vi "Terminal Angle Side view int.vi"(0 "Image":T2, 1 "Search Direction ROI 1":u32(ring)=2 items=["Left to Right", "Right to Left", "Top to Bottom", "Bottom to Top"], 5 "ROI Descriptor":T7 {"Contours"."Type" items=["No Selection", "Point", "Line", "Rectangle", "Oval", "Polygon", "Free", "Annulus", "Unused2", "Unused3", "Broken Line", "Free Hand Line", "Rotated Rectangle"]}, 7 "Edge Options ROI 1":T3={"Edge Polarity"=2, "Kernel Size"=5, "Width"=5, "Minimum Edge Strength"=100.0, "Interpolation Type"=enum."Zero Order", "Data Processing Method"=enum."Average"} {"Edge Polarity" items=["All Edges", "Rising Edges", "Falling Edges"]; "Minimum Edge Strength" format="%.2f"; "Width" step=2; "Kernel Size" step=2}, 9 "Line Options ROI 1":T5={"Number of Lines"=1, "Type"=enum."Best Edge Projection", "Min. Score"=10.0, "Max. Score"=1000.0, "Orientation"=0.0, "Angle Range"=10.0, "Angle Tolerance"=1.0, "Step Size"=3, "Min. SNR (db)"=0.0, "Min. Points (%)"=25.0, "Hough Iterations"=5} {"Min. Points (%)" min=0.0 max=100.0; "Min. SNR (db)" min=0.0; "Max. Score" min=0.0 max=1024.0; "Min. Score" min=0.0 max=1024.0 step=1.0}, 11 "error in (no error)":errorcluster, 12 "OverlayOptions":T1) -> (4 "Angle":sgl, 15 "error out":errorcluster)   [LabVIEW 2019, in "Algorithm.lvclass"]
uses:
  FrameworkOverrides/Algorithm.lvclass
  <vilib>/vision/NI_Vision_Development_Module.lvlib
  <vilib>/vision/Measure.llb/Straight Edge Process.ctl
  <vilib>/vision/Measure.llb/Straight Edge Options.ctl
  <vilib>/vision/Measure.llb/Edge Polarity.ctl
  <vilib>/vision/Measure.llb/Edge Options.ctl
  <vilib>/vision/Image Controls.llb/IMAQ Image.ctl
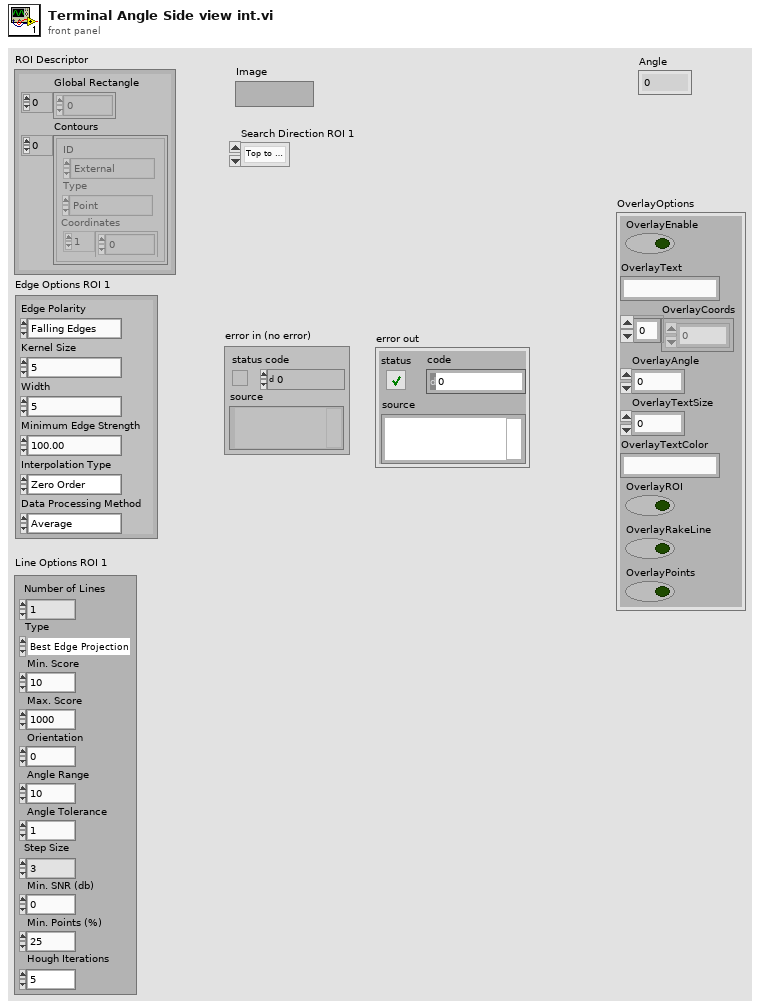
[diagram p1: front panel]
types:
  T1 = cluster{"OverlayEnable":bool, "OverlayText":string, "OverlayCoords":i32[], "OverlayAngle":i32, "OverlayTextSize":i32, "OverlayTextColor":string, "OverlayROI":bool, "OverlayRakeLine":bool, "OverlayPoints":bool}
  T2 = typedef "IMAQ Image.ctl" = refnum<image>
  T3 = typedef "Edge Options.ctl" = cluster{"Edge Polarity":T4, "Kernel Size":u32, "Width":u32, "Minimum Edge Strength":sgl, "Interpolation Type":enum32{"Zero Order", "Bilinear", "Quadratic", "Cubic", "Bilinear Fixed"}, "Data Processing Method":enum32{"Average", "Median"}}
  T4 = typedef "Edge Polarity.ctl" = u32
  T5 = typedef "Straight Edge Options.ctl" = cluster{"Number of Lines":i32, "Type":T6, "Min. Score":dbl, "Max. Score":dbl, "Orientation":dbl, "Angle Range":dbl, "Angle Tolerance":dbl, "Step Size":u32, "Min. SNR (db)":dbl, "Min. Points (%)":dbl, "Hough Iterations":i32}
  T6 = typedef "Straight Edge Process.ctl" = enum32{"First Edge Rake", "Best Edge Rake", "Hough Edge Rake", "First Edge Projection", "Best Edge Projection"}
  T7 = cluster{"Global Rectangle":i32[], "Contours":cluster{"ID":enum32{"External", "Internal"}, "Type":u32, "Coordinates":i32[]}[]}
  T8 = cluster{"Point1 (Pixels)":cluster{"X":sgl, "Y":sgl}, "Point2 (Pixels)":cluster{"X":sgl, "Y":sgl}, "Point1 (Real-World)":cluster{"X":sgl, "Y":sgl}, "Point2 (Real-World)":cluster{"X":sgl, "Y":sgl}, "Angle (Pixel)":dbl, "Angle (Real-World)":dbl, "Score":dbl, "Straightness":dbl, "Average SNR (db)":dbl, "Calibration Valid":bool}[]
  T9 = typedef "Search Line.ctl" = cluster{"Start Point":cluster{"X":sgl, "Y":sgl}, "End Point":cluster{"X":sgl, "Y":sgl}, "Edge Info":T10[], "Edge Map":dbl[], "Calibration Valid":bool}
  T10 = typedef "Edge New.ctl" = cluster{"Location (Pixel)":cluster{"X":sgl, "Y":sgl}, "Location (Real-World)":cluster{"X":sgl, "Y":sgl}, "Distance (Pixel)":dbl, "Distance (Real-World)":dbl, "Strength":dbl, "Noise":dbl, "Rising?":bool}
  T11 = cluster{"Point1 (Pixels)":cluster{"X":sgl, "Y":sgl}, "Point2 (Pixels)":cluster{"X":sgl, "Y":sgl}, "Point1 (Real-World)":cluster{"X":sgl, "Y":sgl}, "Point2 (Real-World)":cluster{"X":sgl, "Y":sgl}, "Angle (Pixel)":dbl, "Angle (Real-World)":dbl, "Score":dbl, "Straightness":dbl, "Average SNR (db)":dbl, "Calibration Valid":bool}
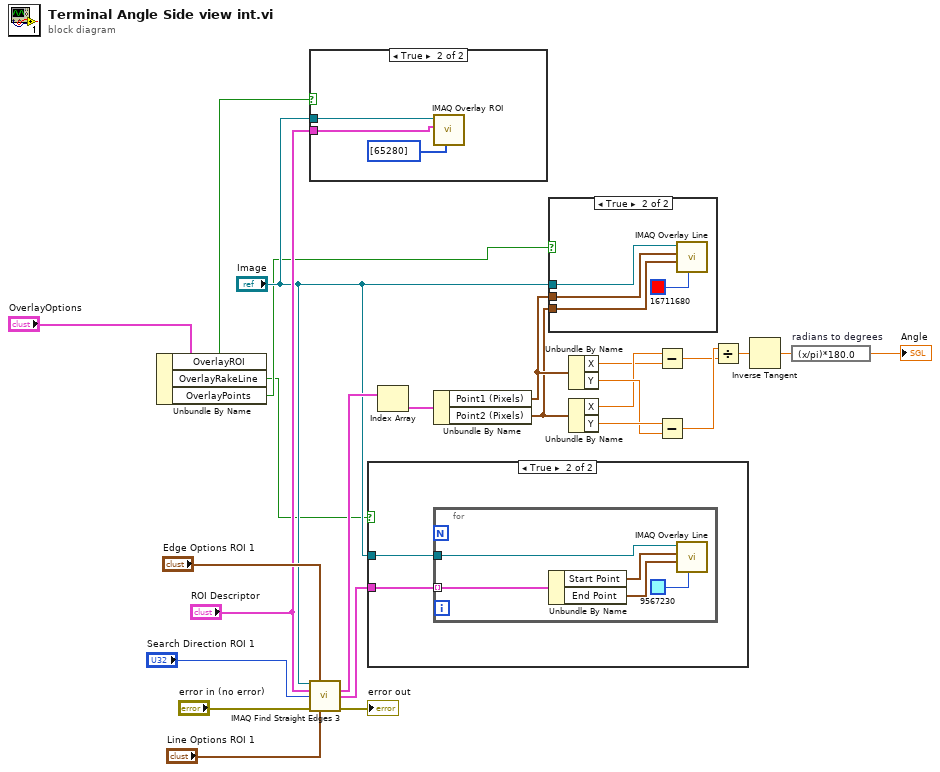
[diagram p0: block diagram]
diagram:
  n1 = Unbundle By Name("OverlayOptions") -> ("OverlayROI"=w3:bool, "OverlayRakeLine"=w1:bool, "OverlayPoints"=w2:bool)
  n2 = case shown="True" w3 {
    tunnel: "ROI Descriptor" -> [_ w28]
    tunnel: "Image" -> [_ w27]
    frame False {
    }
    frame True {
      n3 = call "IMAQ Overlay ROI"("Colors (Green)"=u32[] [65280], "ROI Descriptor"=w28, "Image"=w27) -> ()  [unwired: 7 in, 2 out]
    }
  }
  n4 = call "IMAQ Find Straight Edges 3"("Image"="Image", "Edge Options"="Edge Options ROI 1", "ROI Descriptor"="ROI Descriptor", "Search Direction"="Search Direction ROI 1", "error in (no error)"="error in (no error)", "Line Options"="Line Options ROI 1") -> ("Straight Edges"=w13:T8, "Search Lines Information"=w9:T9[], "error out"=→"error out":errorcluster)  [unwired: 5 in, 2 out]
  n5 = case shown="True" w1 {
    tunnel: w9 -> [_ w30]
    tunnel: "Image" -> [_ w29]
    frame False {
    }
    frame True {
      n6 = for {
        tunnel: w30 -> [w35] mode=indexing
        tunnel: w29 -> [w34]
        n7 = Unbundle By Name(w35) -> ("Start Point"=w33:cluster{"X":sgl, "Y":sgl}, "End Point"=w32:cluster{"X":sgl, "Y":sgl})
        n8 = call "IMAQ Overlay Line"("Color"=u32 9567230, "End Point"=w32, "Start Point"=w33, "Image"=w34) -> ()  [unwired: 6 in, 2 out]
      }
    }
  }
  n9 = Index Array(array=w13) -> (element=w24:T11)  [unwired: 1 in]
  n10 = Unbundle By Name(w24) -> ("Point1 (Pixels)"=w7:cluster{"X":sgl, "Y":sgl}, "Point2 (Pixels)"=w6:cluster{"X":sgl, "Y":sgl})
  n11 = case shown="True" w2 {
    tunnel: w7 -> [_ w39]
    tunnel: w6 -> [_ w38]
    tunnel: "Image" -> [_ w37]
    frame False {
    }
    frame True {
      n12 = call "IMAQ Overlay Line"("Color"=u32 16711680, "End Point"=w38, "Start Point"=w39, "Image"=w37) -> ()  [unwired: 6 in, 2 out]
    }
  }
  n13 = Unbundle By Name(w7) -> ("X"=w20:sgl, "Y"=w22:sgl)
  n14 = Unbundle By Name(w6) -> ("X"=w21:sgl, "Y"=w23:sgl)
  n15 = Subtract(x=w21, y=w20) -> (x-y=w18:sgl)
  n16 = Subtract(x=w23, y=w22) -> (x-y=w19:sgl)
  n17 = Divide(x=w19, y=w18) -> (x/y=w17:sgl)
  n18 = Inverse Tangent(1:w17) -> (0:w15:sgl)
  n19 = expression code="(x/pi)*180.0" "radians to degrees"(w15) -> (→"Angle":sgl)
